vi "PatternMatching.vi"(0 "Image Pixels 1":u32[][](array[numeric]), 5 "Image Pixels 2":u32[][](array[numeric]), 11 "error in (no error)":errorcluster) -> (4 "src":u32[][](array[numeric]), 6 "rect":T1, 8 "score":dbl=1.0, 15 "error out":errorcluster)   [LabVIEW 2014, in "QwaveSys RPi Training Library.lvlib"]
uses:
  <vilib>/Q-Wave Systems/QwaveSys RPi Training Package (Demo)/Addons/QwaveSys RPi Training Library.lvlib
panel:
  out "yB":i32
  out "yT":i32
  out "xR":i32
  out "xL":i32
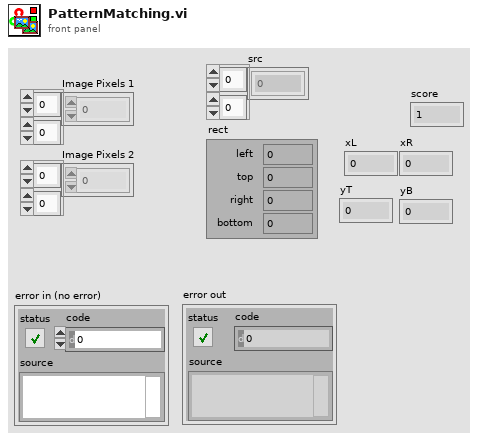
[diagram p1: front panel]
types:
  T1 = cluster{"left":i16, "top":i16, "right":i16, "bottom":i16}
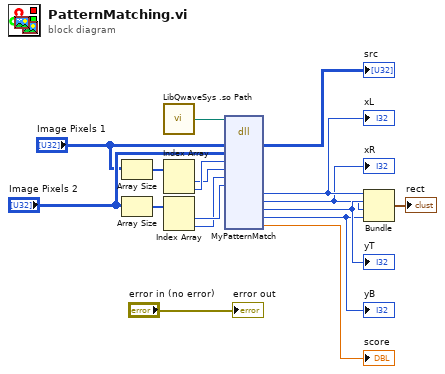
[diagram p0: block diagram]
diagram:
  n1 = Array Size(array="Image Pixels 1") -> (size(s)=w3:i32[])
  n2 = Array Size(array="Image Pixels 2") -> (size(s)=w16:i32[])
  n3 = call <vilib>:"LibQwaveSys .so Path.vi"() -> ("Lib QwaveSys .so Path"=w7:path)  [unwired: 5 in]
  n4 = Index Array(array=w3) -> (element #1=w1:i32, element #2=w2:i32)  [unwired: 2 in]
  n5 = Index Array(array=w16) -> (element #1=w15:i32, element #2=w14:i32)  [unwired: 2 in]
  n6 = dll-call lib="libqwavesys.so" fn="MyPatternMatch"(path in=w7, "src"="Image Pixels 1", "templ"="Image Pixels 2", "src_cols"=w2, "src_rows"=w1, "templ_cols"=w14, "templ_rows"=w15) -> ("src"=→"src":u8[][], "xL"=w13:i32, "xR"=w11:i32, "yT"=w12:i32, "yB"=w10:i32, "score"=→"score":dbl)  [unwired: 13 in, 2 out]
  "xL" <- w13
  "xR" <- w11
  "yT" <- w12
  "yB" <- w10
  n7 = Bundle("xL"=w13, "yT"=w12, "xR"=w11, "yB"=w10) -> (→"rect":cluster{"xL":i32, "yT":i32, "xR":i32, "yB":i32})  [unwired: 1 in]
  "error out" <- "error in (no error)"
